vi "Steganography.vi"() -> ()   [LabVIEW 2015]
uses:
  typedefs/_td MainCluster.ctl
  <vilib>/picture/picture.llb/imagedata.ctl
panel:
  in  "_btn Read Text":bool
  out "O_Text":i16[](array[numeric])
  in  "Sigma (decrypt)":i32=2 min=1 max=100
  in  "_btn Stop":bool
  out "Current Operation":string
  out "Current Iteration":i32=10 min=1 max=100
  in  "Repeat N times":i32=1 min=1 max=100
  in  "_btn Process Image":bool
  out "Decrypted Text":string="Some dummy text to build-in."
  in  "Save File Path":path=path "C:/Users/Kosist/Desktop/Megan_processed.bmp"
  in  "Message Energy":dbl=10.0
  in  "Text to Encrypt":string="Lorem ipsum dolor sit amet, consectetur adipiscing elit, sed do eiusmod tempor incididunt ut labore et dolore magna aliqua. Ut enim ad minim veniam, quis nostrud exercitation ullamco laboris nisi ut aliquip ex ea commodo consequat. Duis aute irure dolor in reprehenderit in voluptate velit esse cillum dolore eu fugiat nulla pariatur. Excepteur sint occaecat cupidatat non proident, sunt in culpa qui officia deserunt mollit anim id est laborum."
  in  "Image Path":path=path "C:/Users/Kosist/Desktop/Megan.bmp"
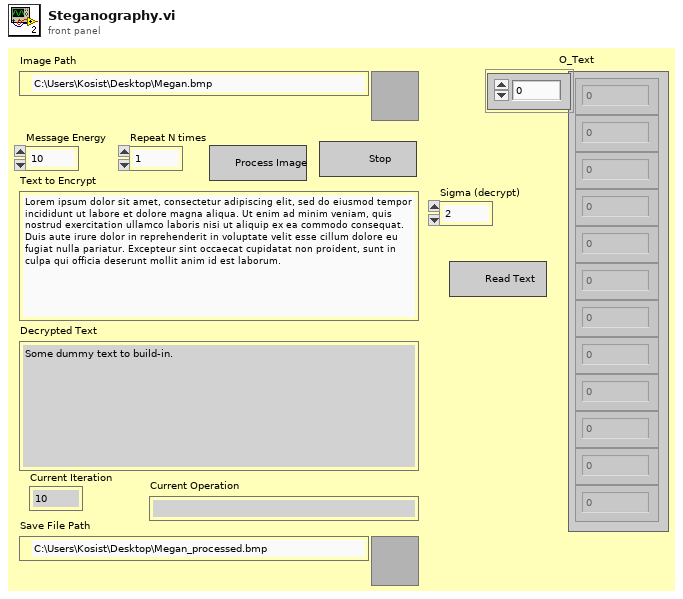
[diagram p1: front panel]
types:
  T1 = enum32{"invalid app kind", "Development System", "Run Time System", "Student Edition", "Embedded LabVIEW", "Evaluation", "Custom"}
  T2 = enum32{"Invalid", "Standard", "Closed", "Hidden", "Minimized", "Maximized"}
  T3 = typedef "_td MainCluster.ctl" = cluster{"SourceImage_FilePath":path, "ProcessedImage_FilePath":path, "Message Energy":dbl, "Text to Encrypt":string, "Decrypted Text":string, "Mixed Pixels Coordinates":i32[][], "Image Data":T4, "Image: Rows":i16, "Image: Columns":i16, "RGB: Red Color":u8[][], "RGB: Green Color":u8[][], "RGB: Blue Color":u8[][], "Required Message Length":i32, "Message Bits Array":u8[], "Mixed RGB Coordinates":i32[], "Repeat N times":i32, "Current Iteration":i32, "Sigma (decrypt)":i32}
  T4 = typedef "imagedata.ctl" = cluster{"image type":i32, "image depth":i32, "image":u8[], "mask":u8[], "colors":u32[], "Rectangle":cluster{"left":i16, "top":i16, "right":i16, "bottom":i16}}
  T5 = cluster{"Core":cluster{"Current VI Reference":refnum<vi>, "Close Panel on Exit?":bool}, "Your Boolean data":bool, "MainCluster":T3}
  T6 = cluster{"Current VI Reference":refnum<vi>, "Close Panel on Exit?":bool}
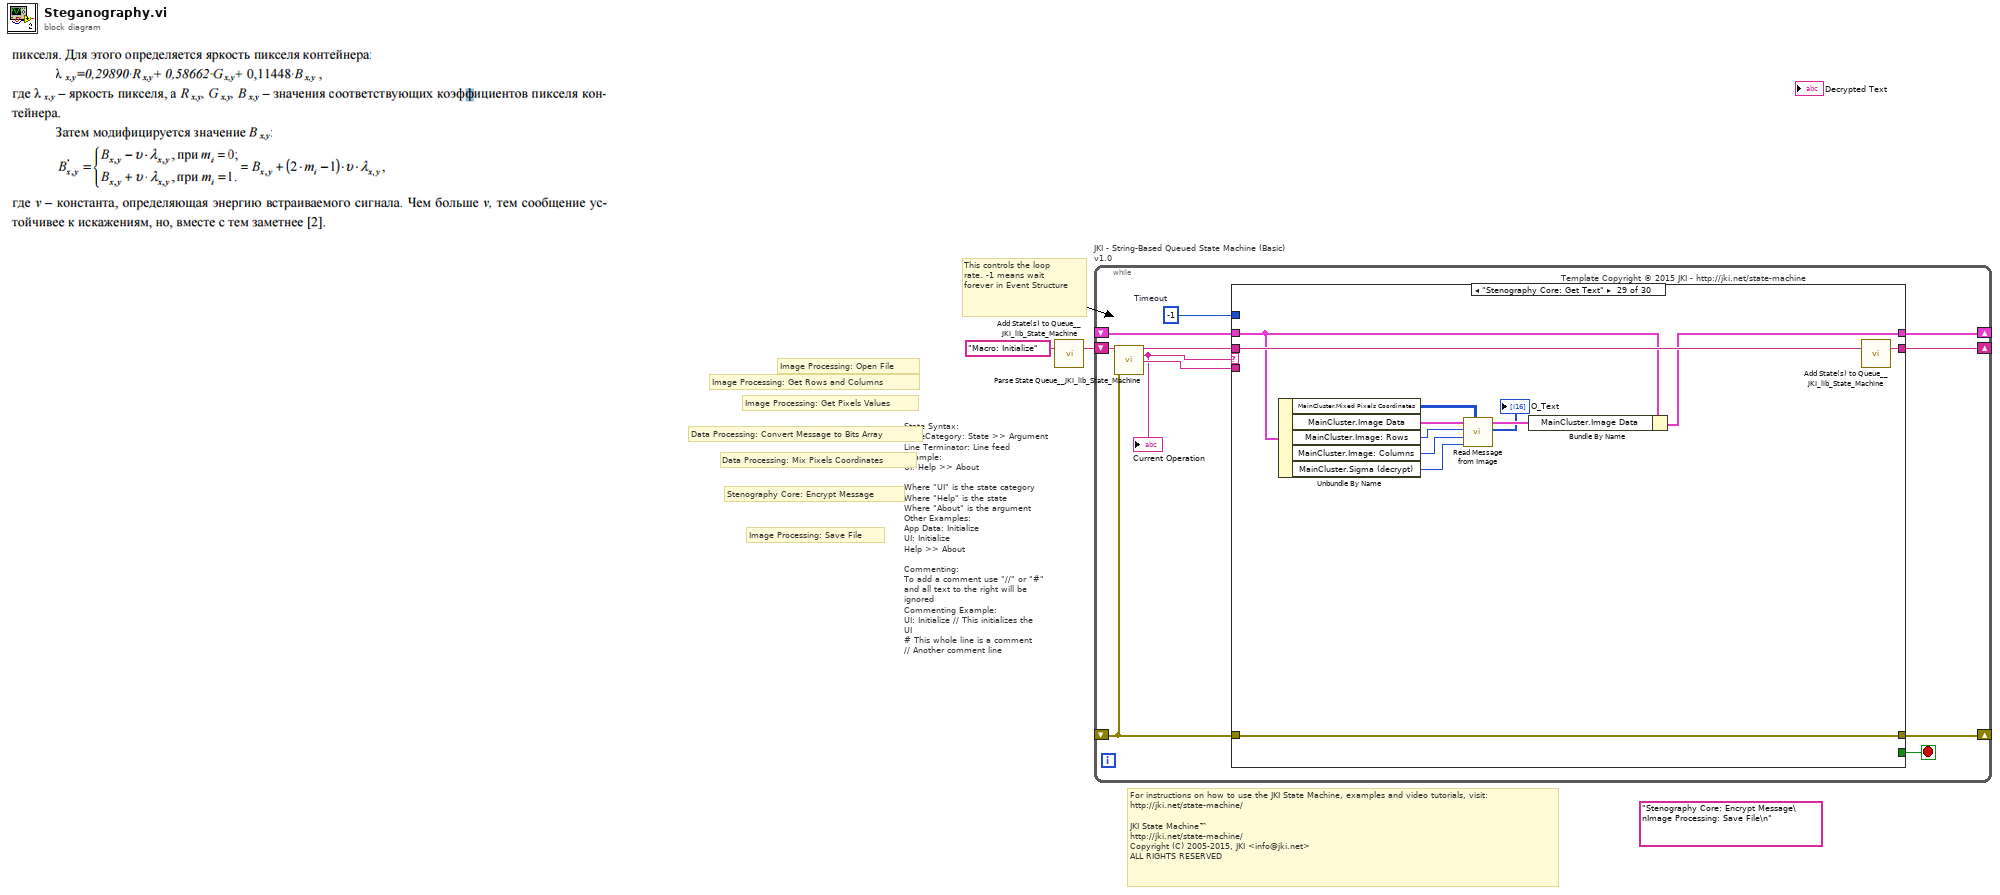
[diagram p0: block diagram]
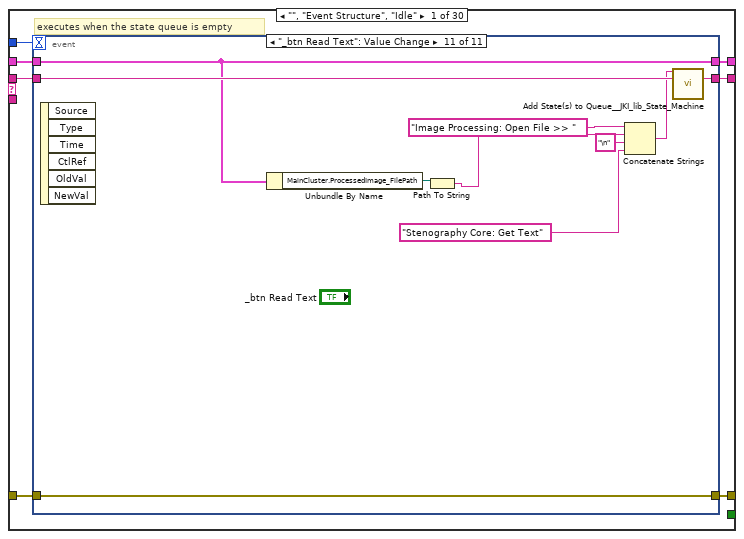
[diagram p2: hidden frame]
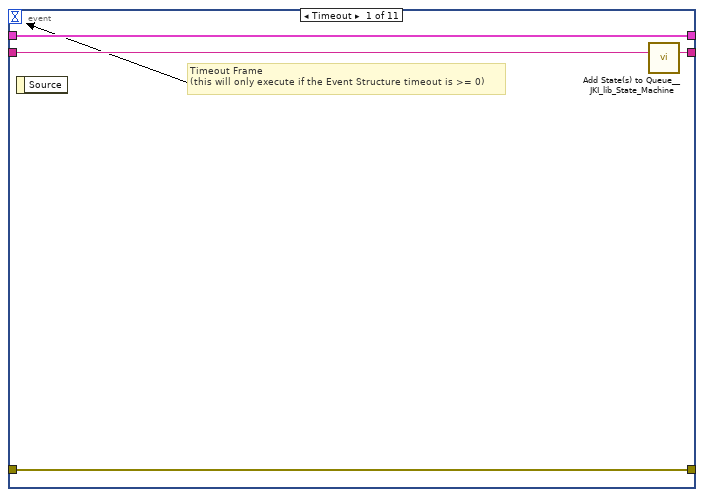
[diagram p3: hidden frame]
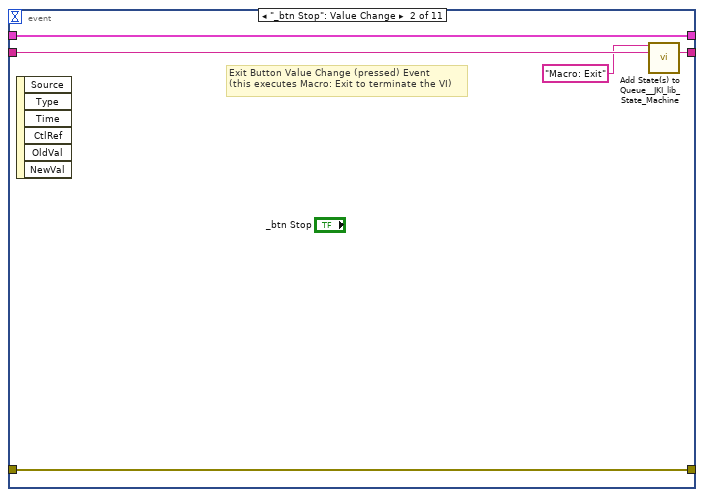
[diagram p4: hidden frame]
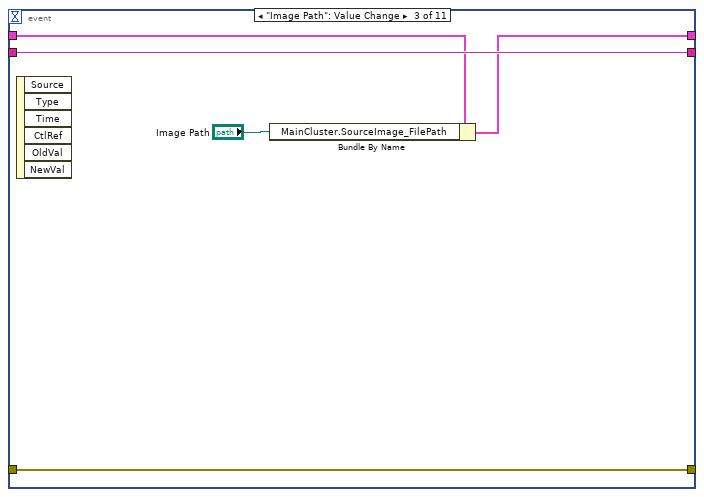
[diagram p5: hidden frame]
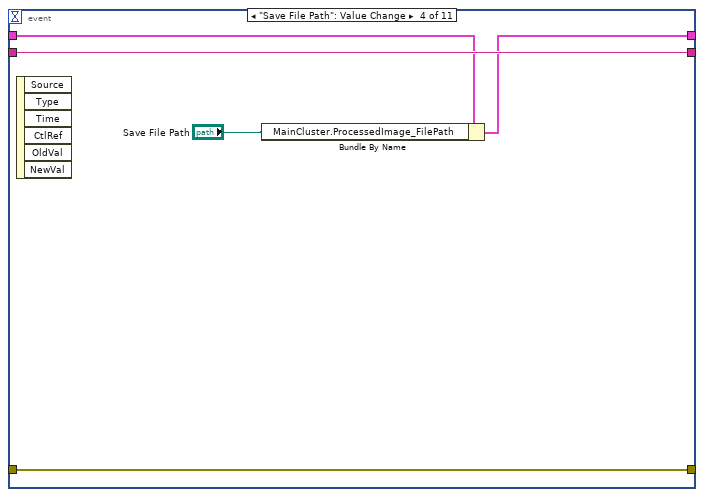
[diagram p6: hidden frame]
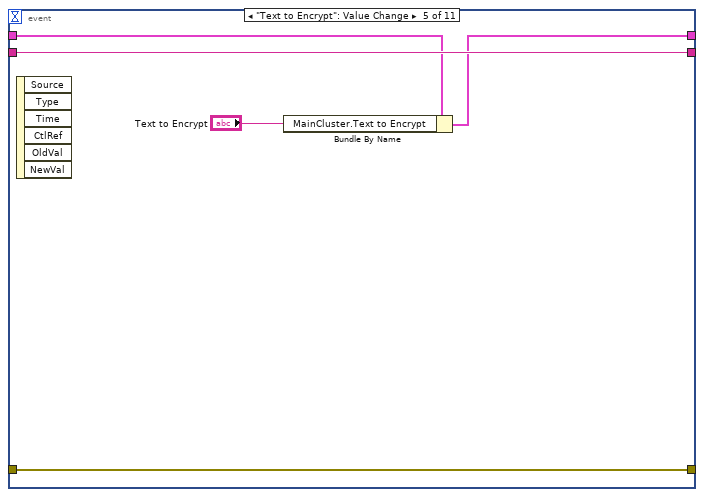
[diagram p7: hidden frame]
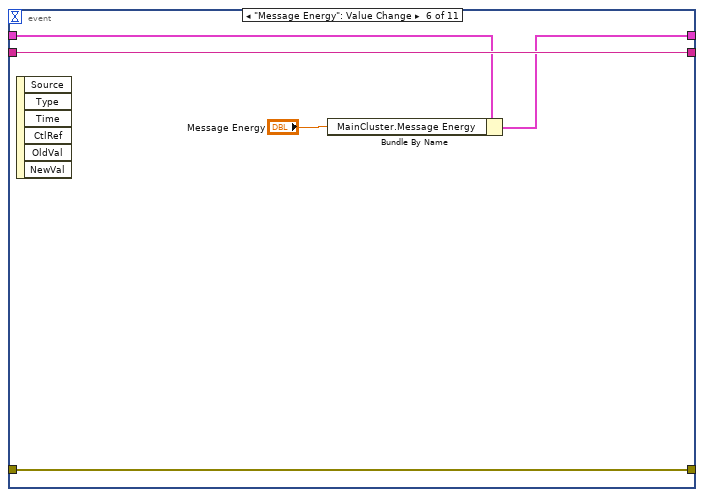
[diagram p8: hidden frame]
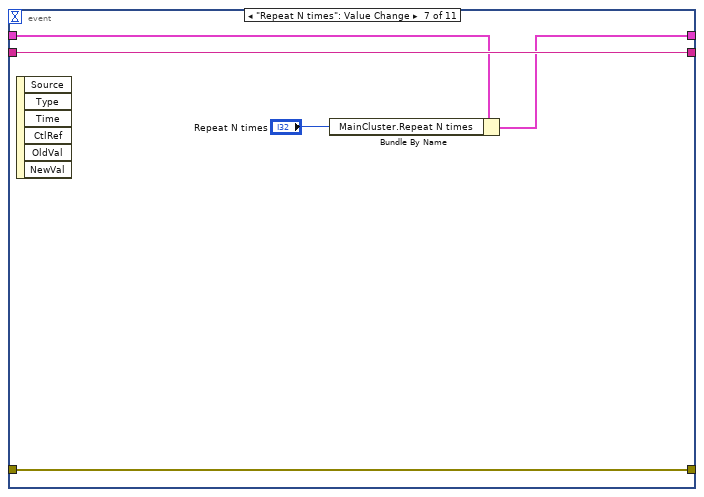
[diagram p9: hidden frame]
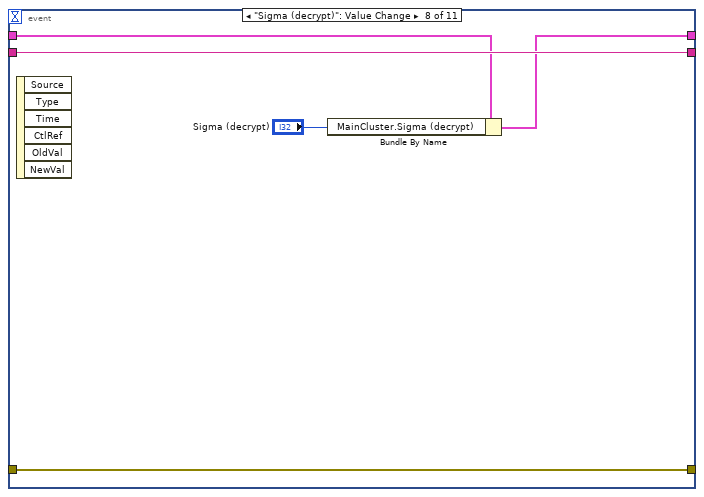
[diagram p10: hidden frame]
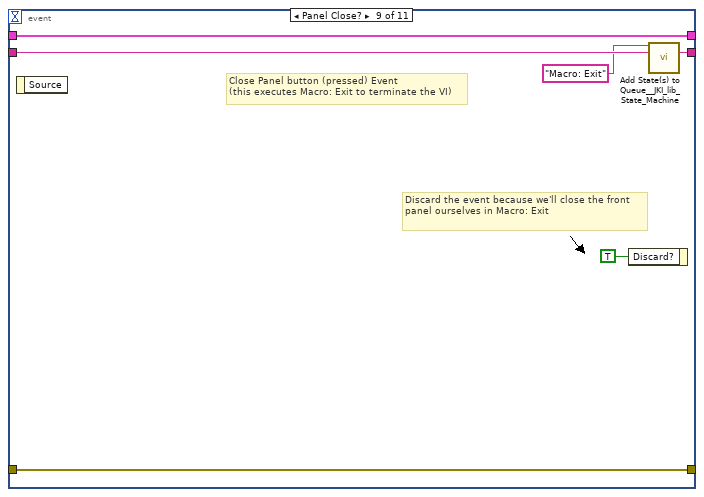
[diagram p11: hidden frame]
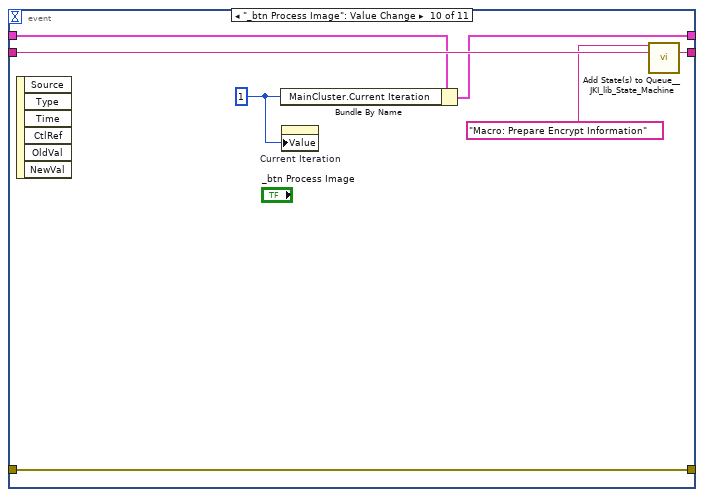
[diagram p12: hidden frame]
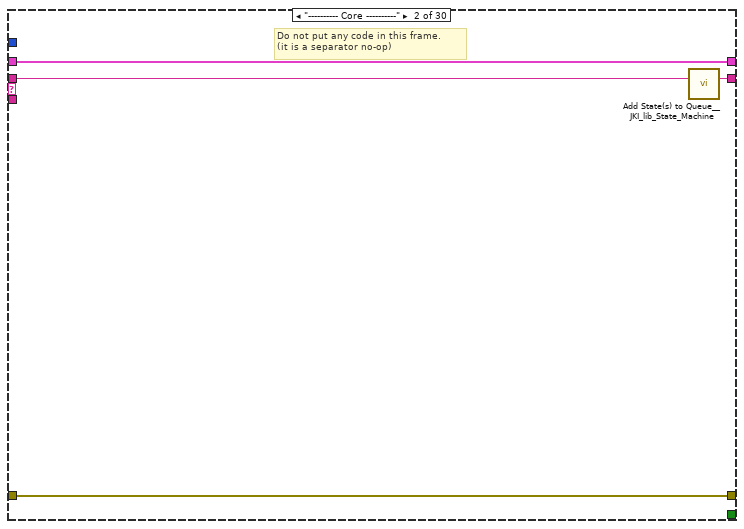
[diagram p13: hidden frame]
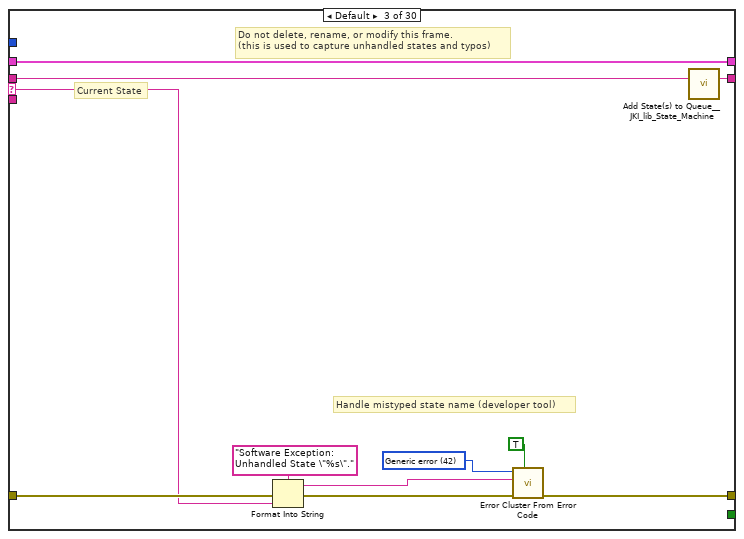
[diagram p14: hidden frame]
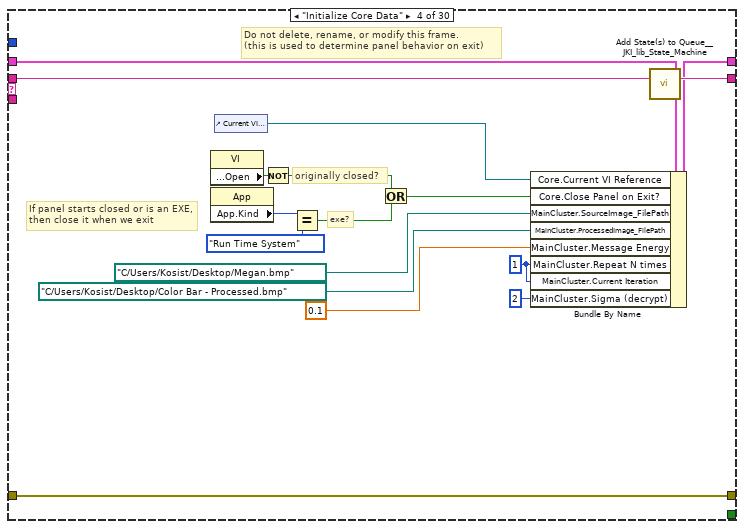
[diagram p15: hidden frame]
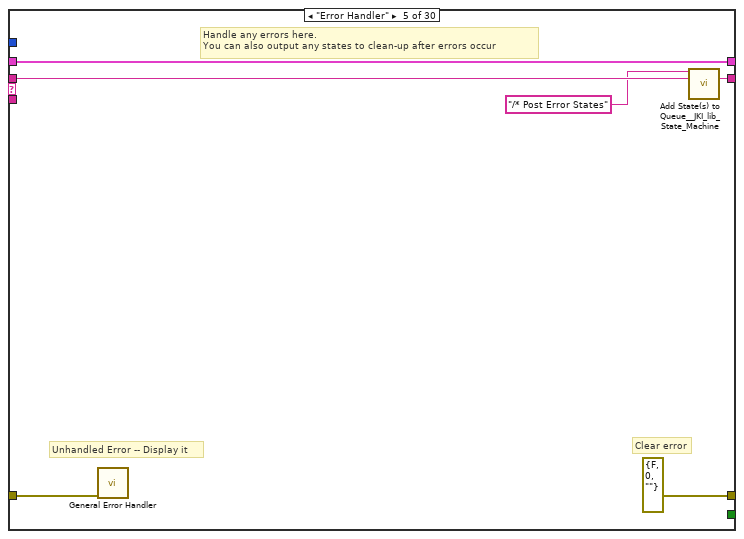
[diagram p16: hidden frame]
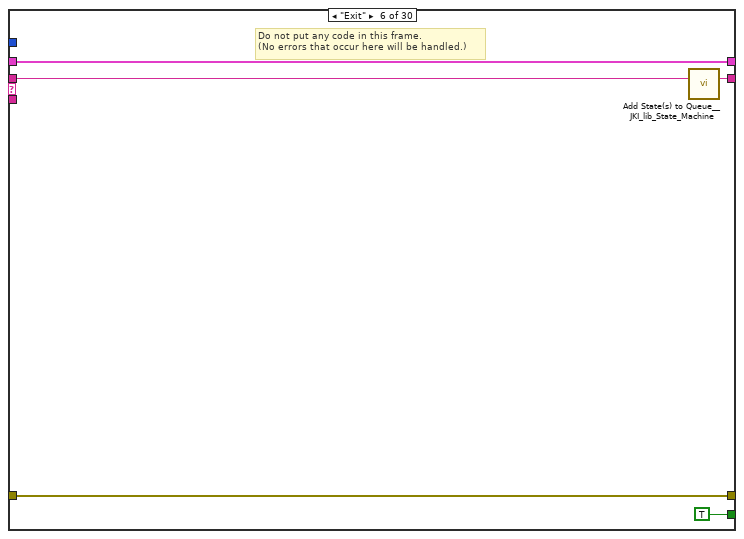
[diagram p17: hidden frame]
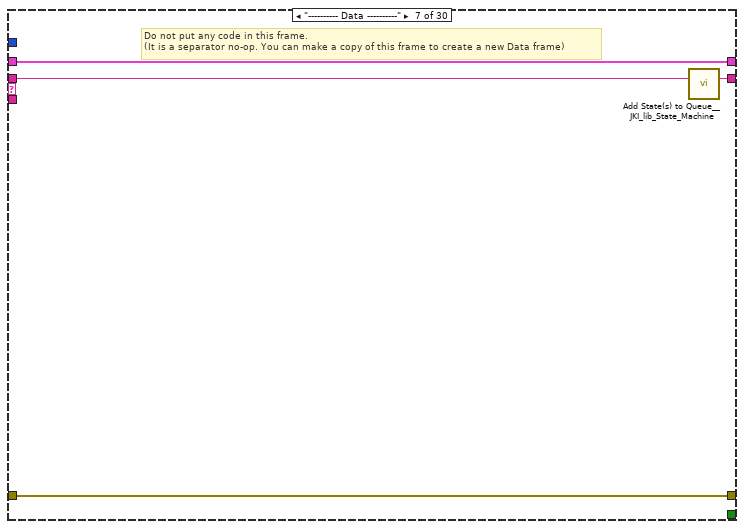
[diagram p18: hidden frame]
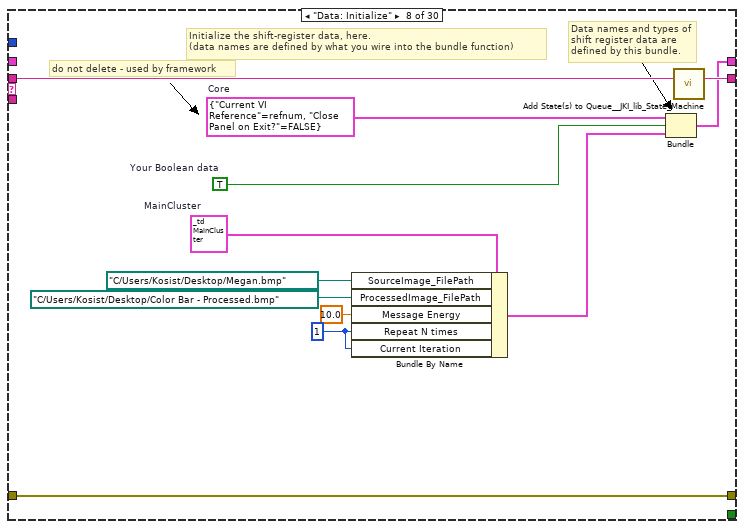
[diagram p19: hidden frame]
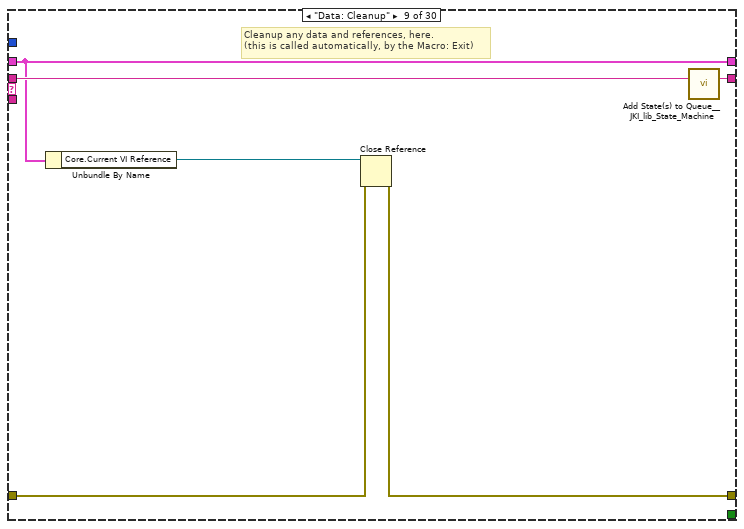
[diagram p20: hidden frame]
diagram:
  (unwired) "Stenography Core: Encrypt Message\nImage Processing: Save File\n"
  # "Image Processing: Save File"
  # "Stenography Core: Encrypt Message"
  # "Data Processing: Mix Pixels Coordinates"
  # "Data Processing: Convert Message to Bits Array"
  # "Image Processing: Get Pixels Values"
  # "Image Processing: Get Rows and Columns"
  # "Image Processing: Open File"
  # "For instructions on how to use the JKI State Machine, examples and video tutorials, visit:\nhttp://jki.net/state-machine/\n\nJKI State Machine™\nhttp://jki.net/state-machine/\nCopyright (C) 2005-2015, JKI <info@jki.net>\nALL RIGHTS RESERVED"
  # "State Syntax:\nStateCategory: State >> Argument\nLine Terminator: Line feed\nExample:\nUI: Help >> About\n\nWhere \"UI\" is the state category\nWhere \"Help\" is the state\nWhere \"About\" is the argument\nOther Examples:\nApp Data: Initialize\nUI: Initialize\nHelp >> About\n\nCommenting:\nTo add a comment use \"//\" or \"#\" and all text to the right will be ignored\nCommenting Example:\nUI: Initialize // This initializes the UI\n# This whole line is a comment\n// Another comment line"
  # "This controls the loop rate. -1 means wait forever in Event Structure"
  n1 = call <vilib>:"Add State(s) to Queue__JKI_lib_State_Machine.vi"("State(s) in (\"\")"="Macro: Initialize") -> ("States Out"=w2:string)  [unwired: 14 in]
  n2 = while "JKI - String-Based Queued State Machine (Basic) v1.0" {
    shift-right: [w7] -> _
    shift-left: _ -> [w6]
    shift-right: [w10] -> _
    shift-left: _ -> [w4]
    shift-right: [w9] -> _
    shift-left: w2 -> [w11]
    stop <- w8 stop-if-true
    w5 = -1  # Timeout
    # "Template Copyright © 2015 JKI - http://jki.net/state-machine"
    n3 = call <vilib>:"Parse State Queue__JKI_lib_State_Machine.vi"("State Queue"=w11, "Error In (no error)"=w4) -> ("Remaining States"=w13:string, "Current State"=w3:string, "Arguments"=w12:string)  [unwired: 11 in]
    "Current Operation" <- w3
    n4 = case shown="\"Stenography Core: Get Text\"" w3 {
      selector: w3 -> [_ _ w87 _ _ _ _ _ _ _ _ _ _ _ _ _ _ _ _ _ _ _ _ _ _ _ _ _ _ _]
      tunnel: w13 -> [w20 w86 w91 w114 w120 w125 w129 w141 w147 w151 w155 w161 w172 w198 w203 w213 w223 w227 w236 w243 w250 w261 w270 w274 w282 w292 w296 w306 w318 w328]
      tunnel: w12 -> [_ _ _ _ _ _ _ _ _ _ _ w156 w166 _ _ _ _ _ w229 _ _ _ _ _ _ _ _ _ _ _]
      tunnel: w6 -> [w18 w83 w89 w105 w117 w123 w126 _ w142 w148 w153 w159 w168 w195 w200 w210 w220 w224 w232 w241 w248 w258 w267 w271 w279 w289 w293 w303 w315 w330]
      tunnel: [w17 w84 w93 w111 errorcluster {"status"=FALSE, "code"=0, "source"=""} ("error out") w122 w127 w138 w143 w149 w152 w157 w169 w196 w201 w211 w221 w225 w233 w237 w247 w259 w268 w272 w280 w290 w294 w304 w316 w319] -> w10
      tunnel: w4 -> [w16 w84 w92 w111 w116 w122 w127 w138 w144 w149 w152 w158 w170 w196 w201 w211 w221 w225 w234 w238 w247 w259 w268 w272 w280 w290 w294 w304 w316 w319]
      tunnel: [w19 w85 w90 w113 w119 w124 w128 w140 w146 w150 w154 w160 w171 w197 w202 w212 w222 w226 w235 w242 w249 w260 w269 w273 w281 w291 w295 w305 w317 w329] -> w9
      tunnel: [_ _ _ _ _ TRUE _ _ _ _ _ _ _ _ _ _ _ _ _ _ _ _ _ _ _ _ _ _ _ _] -> w8
      tunnel: [w15 w83 w89 w112 w117 w123 w126 w139 w142 w148 w153 w159 w168 w195 w200 w210 w220 w224 w231 w241 w246 w257 w266 w271 w278 w285 w293 w298 w314 w326] -> w7
      tunnel: w5 -> [w14 _ _ _ _ _ _ _ _ _ _ _ _ _ _ _ _ _ _ _ _ _ _ _ _ _ _ _ _ _]
      frame "", "Event Structure", "Idle" {
        # "executes when the state queue is empty"
        n5 = event shown="[10] \"_btn Read Text\": Value Change" {
          selector: _ -> [_ _ _ _ _ _ _ _ _ _ _]
          dyn-events: _ -> [_ _ _ _ _ _ _ _ _ _ _]
          timeout: w14 -> [_ _ _ _ _ _ _ _ _ _ _]
          tunnel: w20 -> [w24 w29 w34 w39 w44 w49 w54 w59 w65 w72 w82]
          tunnel: [w23 w28 w34 w39 w44 w49 w54 w59 w64 w71 w81] -> w19
          tunnel: w18 -> [w21 w26 w33 w38 w43 w48 w53 w58 w62 w69 w75]
          tunnel: [w22 w27 w30 w35 w40 w45 w51 w56 w63 w70 w80] -> w17
          tunnel: w16 -> [w22 w27 w30 w35 w40 w45 w51 w56 w63 w70 w80]
          tunnel: [w21 w26 w32 w37 w42 w47 w52 w57 w62 w67 w75] -> w15
          event Timeout {
            # "Timeout Frame\n(this will only execute if the Event Structure timeout is >= 0)"
            n6 = event-data() -> ()  [unwired: 1 in, 1 out]
            n7 = call <vilib>:"Add State(s) to Queue__JKI_lib_State_Machine.vi"("State(s) in (\"\")"=w24) -> ("States Out"=w23:string)  [unwired: 14 in]
          }
          event "_btn Stop": Value Change {
            # "Exit Button Value Change (pressed) Event\n(this executes Macro: Exit to terminate the VI)"
            n8 = event-data() -> ()  [unwired: 1 in, 6 out]
            n9 = call <vilib>:"Add State(s) to Queue__JKI_lib_State_Machine.vi"("State(s) in Front (\"\")"="Macro: Exit", "State(s) in (\"\")"=w29) -> ("States Out"=w28:string)  [unwired: 13 in]
          }
          event "Image Path": Value Change {
            n10 = event-data() -> ()  [unwired: 1 in, 6 out]
            n11 = Bundle By Name(cluster=w33, "MainCluster.SourceImage_FilePath"="Image Path") -> (w32:T5)
          }
          event "Save File Path": Value Change {
            n12 = event-data() -> ()  [unwired: 1 in, 6 out]
            n13 = Bundle By Name(cluster=w38, "MainCluster.ProcessedImage_FilePath"="Save File Path") -> (w37:T5)
          }
          event "Text to Encrypt": Value Change {
            n14 = event-data() -> ()  [unwired: 1 in, 6 out]
            n15 = Bundle By Name(cluster=w43, "MainCluster.Text to Encrypt"="Text to Encrypt") -> (w42:T5)
          }
          event "Message Energy": Value Change {
            n16 = event-data() -> ()  [unwired: 1 in, 6 out]
            n17 = Bundle By Name(cluster=w48, "MainCluster.Message Energy"="Message Energy") -> (w47:T5)
          }
          event "Repeat N times": Value Change {
            n18 = event-data() -> ()  [unwired: 1 in, 6 out]
            n19 = Bundle By Name(cluster=w53, "MainCluster.Repeat N times"="Repeat N times") -> (w52:T5)
          }
          event "Sigma (decrypt)": Value Change {
            n20 = event-data() -> ()  [unwired: 1 in, 6 out]
            n21 = Bundle By Name(cluster=w58, "MainCluster.Sigma (decrypt)"="Sigma (decrypt)") -> (w57:T5)
          }
          event Panel Close? {
            # "Discard the event because we'll close the front panel ourselves in Macro: Exit"
            # "Close Panel button (pressed) Event\n(this executes Macro: Exit to terminate the VI)"
            n22 = event-data() -> ()  [unwired: 1 in, 1 out]
            n23 = event-data("Discard?"=TRUE) -> ()  [unwired: 1 in, 1 out]
            n24 = call <vilib>:"Add State(s) to Queue__JKI_lib_State_Machine.vi"("State(s) in Front (\"\")"="Macro: Exit", "State(s) in (\"\")"=w65) -> ("States Out"=w64:string)  [unwired: 13 in]
          }
          event "_btn Process Image": Value Change {
            w66 = 1 ("MainCluster.Current Iteration")
            n25 = event-data() -> ()  [unwired: 1 in, 6 out]
            n26 = Bundle By Name(cluster=w69, "MainCluster.Current Iteration"=w66) -> (w67:T5)
            n27 = property on="Current Iteration" class="DigNum (strict)"("Value"=w66) -> ()  [unwired: 2 in, 2 out]
            n28 = call <vilib>:"Add State(s) to Queue__JKI_lib_State_Machine.vi"("State(s) in Front (\"\")"="Macro: Prepare Encrypt Information", "State(s) in (\"\")"=w72) -> ("States Out"=w71:string)  [unwired: 13 in]
          }
          event "_btn Read Text": Value Change {
            n29 = event-data() -> ()  [unwired: 1 in, 6 out]
            n30 = Unbundle By Name(w75) -> ("MainCluster.ProcessedImage_FilePath"=w79:path)
            n31 = Path To String(path=w79) -> (string=w77:string)
            n32 = Concatenate Strings("Image Processing: Open File >> ", w77, "\n" ("string"), "Stenography Core: Get Text") -> (w73:string)
            n33 = call <vilib>:"Add State(s) to Queue__JKI_lib_State_Machine.vi"("State(s) in Front (\"\")"=w73, "State(s) in (\"\")"=w82) -> ("States Out"=w81:string)  [unwired: 13 in]
          }
        }
      }
      frame "---------- Core ----------" {
        # "Do not put any code in this frame.\n(it is a separator no-op)"
        n34 = call <vilib>:"Add State(s) to Queue__JKI_lib_State_Machine.vi"("State(s) in (\"\")"=w86) -> ("States Out"=w85:string)  [unwired: 14 in]
      }
      frame Default {
        w96 = 42 items=["No error", "Argument error", "Memory is full", "Out of zone", "End of file", "File already open", "Generic file I/O error", "File not found", "File permission error", "Disk is full", "Duplicate path", "Too many files open", "System feature not enabled", "Resource file not found", "Cannot add resource", "Resource not found", "Image not found", "Image memory error", "Pen does not exist", "Config type invalid", "Config token not found", "Config parse error", "Config memory error", "Bad external code format", "Bad external code offset", "External code not present", "Null window", "Destroy window error", "Null menu", "Print aborted", "Bad print record", "Print driver error", "Windows error during printing", "Memory error during printing", "Print dialog error", "Generic print error", "Invalid device refnum", "Device not found", "Device parameter error", "Device unit error", "Cannot open device", "Device call aborted", "Generic error", "Cancelled by user", "Object ID too low", "Object ID too high", "Object not in heap", "Unknown heap", "Unknown object (invalid DefProc)", "Unknown object (DefProc not in table)", "Message out of range", "Invalid (null) method", "Unknown message", "Manager call not supported", "Bad address", "Network operation in progress", "Network operation timed out", "Connection is busy", "Network attribute not supported", "Network error", "Address in use", "System out of memory", "Connection aborted", "Connection refused", "Not connected", "Already connected", "Connection closed", "Initialization error (interapplication manager)", "Bad occurrence", "Wait on unbound occurrence handler", "Occurrence queue overflow", "Datalog type conflict", "Unused", "Unrecognized type (interapplication manager)", "Memory corrupt", "Failed to make temporary DLL", "Old CIN version", "Drag socket not found", "Failed to load drop-object", "Failed to register OLE object", "Failed to release OLE object", "Format specifier type mismatch", "Unknown format specifier", "Too few format specifiers", "Too many format specifiers", "Scan failed", "Newer CIN version", "Error converting to variant", "Runtime menu error", "Password tampered", "Variant attribute not found", "Incompatible variant data type", "Event data is not available", "Event Store is not present", "Occurrence is not found", "Event Queue is not created", "Event info is not available", "Refnum passed is NULL", "Error retrieving Class GUID", "Error retrieving CoClass GUID", "Error retrieving TypeLib GUID.", "Bad built application magic bytes.", "Specific driver is different from the specific driver associated with the Logical Name.", "There is no session opened to the class driver.", "Max Error", "MAX - Error with config objects", "MAX - Error loading configuration", "MAX - Group not supported"]
        # "Current State"
        # "Do not delete, rename, or modify this frame.\n(this is used to capture unhandled states and typos)"
        # "Handle mistyped state name (developer tool)"
        n35 = Format Into String(format string="Software Exception: Unhandled State \"%s\"." ("message"), error in=w92, w87) -> (resulting string=w95:string, error out=w94:errorcluster)  [unwired: 1 in]
        n36 = call <vilib>:"Error Cluster From Error Code.vi"("show call chain? (False)"=TRUE, "error in (no error)"=w94, "error message (\"\")"=w95, "error code (0)"=w96) -> ("error out"=w93:errorcluster)  [unwired: 5 in]
        n37 = call <vilib>:"Add State(s) to Queue__JKI_lib_State_Machine.vi"("State(s) in (\"\")"=w91) -> ("States Out"=w90:string)  [unwired: 14 in]
      }
      frame "Initialize Core Data" {
        w99 = 1 ("MainCluster.Repeat N times")
        # "Do not delete, rename, or modify this frame.\n(this is used to determine panel behavior on exit)"
        # "originally closed?"
        # "exe?"
        # "If panel starts closed or is an EXE, then close it when we exit"
        n38 = property class="VI"() -> ("Front Panel.Open"=w110:bool)  [unwired: 2 in, 2 out]
        n39 = property class="App"() -> ("App.Kind"=w109:T1)  [unwired: 2 in, 2 out]
        n40 = control-ref of="Current VI Reference"() -> (w103:refnum<vi>)
        n41 = Not(x=w110) -> (.not. x?=w107:bool)
        n42 = Equal?(x=w109, y=T1."Run Time System" ("Application:Kind")) -> (x = y?=w106:bool)
        n43 = Or(x=w107, y=w106) -> (x .or. y?=w104:bool)
        n44 = Bundle By Name(cluster=w105, "Core.Current VI Reference"=w103, "Core.Close Panel on Exit?"=w104, "MainCluster.SourceImage_FilePath"=path "C:/Users/Kosist/Desktop/Megan.bmp" ("_td MainCluster.SourceImage_FilePath"), "MainCluster.ProcessedImage_FilePath"=path "C:/Users/Kosist/Desktop/Color Bar - Processed.bmp" ("_td MainCluster.SourceImage_FilePath"), "MainCluster.Message Energy"=0.1 ("_td MainCluster.Message Energy"), "MainCluster.Repeat N times"=w99, "MainCluster.Current Iteration"=w99, "MainCluster.Sigma (decrypt)"=2) -> (w112:T5)
        n45 = call <vilib>:"Add State(s) to Queue__JKI_lib_State_Machine.vi"("State(s) in (\"\")"=w114) -> ("States Out"=w113:string)  [unwired: 14 in]
      }
      frame "Error Handler" {
        # "Unhandled Error -- Display it"
        # "Handle any errors here.\nYou can also output any states to clean-up after errors occur"
        # "Clear error"
        n46 = call <vilib>:"General Error Handler.vi"("error in (no error)"=w116) -> ()  [unwired: 10 in, 5 out]
        n47 = call <vilib>:"Add State(s) to Queue__JKI_lib_State_Machine.vi"("State(s) in Front (\"\")"="/* Post Error States", "State(s) in (\"\")"=w120) -> ("States Out"=w119:string)  [unwired: 13 in]
      }
      frame "Exit" {
        # "Do not put any code in this frame.\n(No errors that occur here will be handled.)"
        n48 = call <vilib>:"Add State(s) to Queue__JKI_lib_State_Machine.vi"("State(s) in (\"\")"=w125) -> ("States Out"=w124:string)  [unwired: 14 in]
      }
      frame "---------- Data ----------" {
        # "Do not put any code in this frame.\n(It is a separator no-op. You can make a copy of this frame to create a new Data frame)"
        n49 = call <vilib>:"Add State(s) to Queue__JKI_lib_State_Machine.vi"("State(s) in (\"\")"=w129) -> ("States Out"=w128:string)  [unwired: 14 in]
      }
      frame "Data: Initialize" {
        w130 = 1 ("Repeat N times")
        w135 = T3 {"SourceImage_FilePath"=path "", "ProcessedImage_FilePath"=path "", "Message Energy"=0.0, "Text to Encrypt"="", "Decrypted Text"="", "Mixed Pixels Coordinates"=[], "Image Data"={"image type"=0, "image depth"=0, "image"=[], "mask"=[], "colors"=[], "Rectangle"={"left"=0, "top"=0, "right"=0, "bottom"=0}}, "Image: Rows"=0, "Image: Columns"=0, "RGB: Red Color"=[], "RGB: Green Color"=[], "RGB: Blue Color"=[], "Required Message Length"=0, "Message Bits Array"=[], "Mixed RGB Coordinates"=[], "Repeat N times"=0, "Current Iteration"=0, "Sigma (decrypt)"=2}  # MainCluster
        w136 = T6 {"Current VI Reference"=refnum, "Close Panel on Exit?"=FALSE}  # Core
        w137 = TRUE  # Your Boolean data
        # "do not delete - used by framework"
        # "Data names and types of shift register data are defined by this bundle."
        # "Initialize the shift-register data, here.\n(data names are defined by what you wire into the bundle function)"
        n50 = Bundle By Name(cluster=w135, "SourceImage_FilePath"=path "C:/Users/Kosist/Desktop/Megan.bmp" ("Image Path"), "ProcessedImage_FilePath"=path "C:/Users/Kosist/Desktop/Color Bar - Processed.bmp" ("Save File Path"), "Message Energy"=10.0, "Repeat N times"=w130, "Current Iteration"=w130) -> (w134:T3)
        n51 = Bundle("Core"=w136, "Your Boolean data"=w137, "MainCluster"=w134) -> (w139:T5)  [unwired: 1 in]
        n52 = call <vilib>:"Add State(s) to Queue__JKI_lib_State_Machine.vi"("State(s) in (\"\")"=w141) -> ("States Out"=w140:string)  [unwired: 14 in]
      }
      frame "Data: Cleanup" {
        # "Cleanup any data and references, here.\n(this is called automatically, by the Macro: Exit)"
        n53 = Unbundle By Name(w142) -> ("Core.Current VI Reference"=w145:refnum<vi>)
        n54 = Close Reference(reference=w145, error in (no error)=w144) -> (error out=w143:errorcluster)
        n55 = call <vilib>:"Add State(s) to Queue__JKI_lib_State_Machine.vi"("State(s) in (\"\")"=w147) -> ("States Out"=w146:string)  [unwired: 14 in]
      }
      frame "---------- UI ----------" {
        # "Do not put any code in this frame.\n(It is a separator no-op. You can make a copy of this frame to create a new UI frame)"
        n56 = call <vilib>:"Add State(s) to Queue__JKI_lib_State_Machine.vi"("State(s) in (\"\")"=w151) -> ("States Out"=w150:string)  [unwired: 14 in]
      }
      frame "UI: Initialize" {
        # "Initialize the User Interface, here.\n(this is called automatically, by the Macro: Init)"
        n57 = call <vilib>:"Add State(s) to Queue__JKI_lib_State_Machine.vi"("State(s) in (\"\")"=w155) -> ("States Out"=w154:string)  [unwired: 14 in]
      }
      frame "UI: Cursor Set" {
        # "Argument"
        # "Set and Unset Cursor Busy.\n(Usage: \"UI: Cursor Set >> Busy|Idle\")"
        n58 = case shown="\"Idle\", Default" w156 {
          tunnel: w158 -> [w163 w165]
          tunnel: [w162 w164] -> w157
          frame "Idle", Default {
            n59 = call <vilib>:"Unset Busy.vi"("error in (no error)"=w163) -> ("error out"=w162:errorcluster)  [unwired: 10 in]
          }
          frame "Busy" {
            n60 = call <vilib>:"Set Busy.vi"("error in (no error)"=w165) -> ("error out"=w164:errorcluster)  [unwired: 9 in, 1 out]
          }
        }
        n61 = call <vilib>:"Add State(s) to Queue__JKI_lib_State_Machine.vi"("State(s) in (\"\")"=w161) -> ("States Out"=w160:string)  [unwired: 14 in]
      }
      frame "UI: Front Panel State" {
        # "Argument"
        # "Set Front Panel Open or Closed\n(Usage: \"UI: Front Panel State >> Open|Close\")"
        n62 = Unbundle By Name(w168) -> ("Core.Current VI Reference"=w167:refnum<vi>)
        n63 = case shown="\"Open\", Default" w166 {
          tunnel: w170 -> [w176 w189]
          tunnel: [w178 w190] -> w169
          tunnel: w167 -> [w177 w187]
          frame "Open", Default {
            n64 = property class="VI"(reference=w177, error in=w176) -> (reference out=w174:refnum<vi>, error out=w175:errorcluster, "Front Panel.Open"=w173:bool)
            n65 = case shown="False" w173 {
              tunnel: [w181 w184] -> w178
              tunnel: w175 -> [w180 w184]
              tunnel: w174 -> [w179 _]
              frame False {
                n66 = invoke class="VI" method="FP.Open"(reference=w179, error in=w180, "Activate"=TRUE, "State"=T2."Standard") -> (error out=w181:errorcluster)  [unwired: 1 in, 4 out]
              }
              frame True {
              }
            }
          }
          frame "Close" {
            n67 = property class="VI"(reference=w187, error in=w189) -> (reference out=w186:refnum<vi>, error out=w188:errorcluster, "Front Panel.Open"=w185:bool)
            n68 = case shown="True" w185 {
              tunnel: [w191 w194] -> w190
              tunnel: w188 -> [w191 w193]
              tunnel: w186 -> [_ w192]
              frame False {
              }
              frame True {
                n69 = invoke class="VI" method="FP.Close"(reference=w192, error in=w193) -> (error out=w194:errorcluster)  [unwired: 1 in, 2 out]
              }
            }
          }
        }
        n70 = call <vilib>:"Add State(s) to Queue__JKI_lib_State_Machine.vi"("State(s) in (\"\")"=w172) -> ("States Out"=w171:string)  [unwired: 14 in]
      }
      frame "---------- Macro ----------" {
        # "Do not put any code in this frame.\n(It is a separator no-op. You can make a copy of this frame to create a new Macro frame)"
        n71 = call <vilib>:"Add State(s) to Queue__JKI_lib_State_Machine.vi"("State(s) in (\"\")"=w198) -> ("States Out"=w197:string)  [unwired: 14 in]
      }
      frame "Macro: Initialize" {
        w199 = "Data: Initialize\nInitialize Core Data\nUI: Initialize\nUI: Front Panel State >> Open"  # Data: Initialize Initialize Core Data UI: Initialize UI: Front Panel State >> Open
        # "Initialization Macro\n(This is called once, when the VI starts)"
        n72 = call <vilib>:"Add State(s) to Queue__JKI_lib_State_Machine.vi"("State(s) in Front (\"\")"=w199, "State(s) in (\"\")"=w203) -> ("States Out"=w202:string)  [unwired: 13 in]
      }
      frame "Macro: Prepare Encrypt Information" {
        n73 = Unbundle By Name(w210) -> ("MainCluster.SourceImage_FilePath"=w209:path)
        n74 = Path To String(path=w209) -> (string=w207:string)
        n75 = Concatenate Strings("Image Processing: Open File >> ", w207, "\n" ("string"), "Image Processing: Get Rows and Columns\nImage Processing: Get Pixels Values\nData Processing: Convert Message to Bits Array\nData Processing: Mix Pixels Coordinates\nStenography Core: Encrypt Message\nStenography Core: Iteration Control") -> (w204:string)
        n76 = call <vilib>:"Add State(s) to Queue__JKI_lib_State_Machine.vi"("State(s) in Front (\"\")"=w204, "State(s) in (\"\")"=w213) -> ("States Out"=w212:string)  [unwired: 13 in]
      }
      frame "Macro: Exit" {
        # "Exit Macro\n(This is called once, when the VI exits)"
        n77 = Unbundle By Name(w220) -> ("Core.Close Panel on Exit?"=w219:bool)
        n78 = Select(t="UI: Front Panel State >> Close", s=w219, f="") -> (s? t:f=w216:string)
        n79 = call <vilib>:"Add State(s) to Queue__JKI_lib_State_Machine.vi"("State(s) in (\"\")"=w216, "State(s) at Back (\"\")"="Data: Cleanup\nExit") -> ("States Out"=w214:string)  [unwired: 13 in]
        n80 = call <vilib>:"Add State(s) to Queue__JKI_lib_State_Machine.vi"("State(s) in Front (\"\")"=w214, "State(s) in (\"\")"=w223) -> ("States Out"=w222:string)  [unwired: 13 in]
      }
      frame "---------- Image Processing ----------" {
        # "Template Separator\n(You can make a copy of, or modify, this frame)"
        n81 = call <vilib>:"Add State(s) to Queue__JKI_lib_State_Machine.vi"("State(s) in (\"\")"=w227) -> ("States Out"=w226:string)  [unwired: 14 in]
      }
      frame "Image Processing: Open File" {
        n82 = String To Path(string=w229) -> (path=w228:path)
        n83 = call <vilib>:"Read BMP File.vi"("error in (no error)"=w234, "path to BMP file"=w228) -> ("error out"=w233:errorcluster, "image data"=w230:T4)  [unwired: 7 in, 1 out]
        n84 = Bundle By Name(cluster=w232, "MainCluster.Image Data"=w230) -> (w231:T5)
        n85 = call <vilib>:"Add State(s) to Queue__JKI_lib_State_Machine.vi"("State(s) in (\"\")"=w236) -> ("States Out"=w235:string)  [unwired: 14 in]
      }
      frame "Image Processing: Save File" {
        n86 = Unbundle By Name(w241) -> ("MainCluster.ProcessedImage_FilePath"=w240:path, "MainCluster.Image Data"=w239:T4)
        n87 = call <vilib>:"Write BMP File.vi"("error in (no error)"=w238, "image data"=w239, "path to BMP file"=w240) -> ("error out"=w237:errorcluster)  [unwired: 7 in, 1 out]
        n88 = call <vilib>:"Add State(s) to Queue__JKI_lib_State_Machine.vi"("State(s) in (\"\")"=w243) -> ("States Out"=w242:string)  [unwired: 14 in]
      }
      frame "Image Processing: Get Rows and Columns" {
        n89 = Unbundle By Name(w248) -> ("MainCluster.Image Data.Rectangle.bottom"=w245:i16, "MainCluster.Image Data.Rectangle.right"=w244:i16)
        n90 = Bundle By Name(cluster=w248, "MainCluster.Image: Rows"=w245, "MainCluster.Image: Columns"=w244) -> (w246:T5)
        n91 = call <vilib>:"Add State(s) to Queue__JKI_lib_State_Machine.vi"("State(s) in (\"\")"=w250) -> ("States Out"=w249:string)  [unwired: 14 in]
      }
      frame "Image Processing: Get Pixels Values" {
        n92 = Unbundle By Name(w258) -> ("MainCluster.Image Data.image"=w256:u8[], "MainCluster.Image Data.Rectangle.bottom"=w255:i16, "MainCluster.Image Data.Rectangle.right"=w254:i16)
        n93 = call "Get RGB Pixels Values.vi"("I_Number of columns"=w254, "I_Number of rows"=w255, "I_Image Data"=w256) -> ("O_RGB: Blue Color"=w251:u8[][], "O_RGB: Green Color"=w252:u8[][], "O_RGB: Red Color"=w253:u8[][])  [unwired: 6 in]
        n94 = Bundle By Name(cluster=w258, "MainCluster.RGB: Red Color"=w253, "MainCluster.RGB: Green Color"=w252, "MainCluster.RGB: Blue Color"=w251) -> (w257:T5)
        n95 = call <vilib>:"Add State(s) to Queue__JKI_lib_State_Machine.vi"("State(s) in (\"\")"=w261) -> ("States Out"=w260:string)  [unwired: 14 in]
      }
      frame "Image Processing: Pixels Values to Image" {
        n96 = Unbundle By Name(w267) -> ("MainCluster.RGB: Red Color"=w265:u8[][], "MainCluster.RGB: Green Color"=w264:u8[][], "MainCluster.RGB: Blue Color"=w263:u8[][])
        n97 = call "RGB Pixels Values to Image.vi"("I_RGB: Blue Color"=w263, "I_RGB: Green Color"=w264, "I_RGB: Red Color"=w265) -> ("O_Image Data"=w262:u8[])  [unwired: 8 in]
        n98 = Bundle By Name(cluster=w267, "MainCluster.Image Data.image"=w262) -> (w266:T5)
        n99 = call <vilib>:"Add State(s) to Queue__JKI_lib_State_Machine.vi"("State(s) in (\"\")"=w270) -> ("States Out"=w269:string)  [unwired: 14 in]
      }
      frame "---------- Data Processing ----------" {
        # "Template Separator\n(You can make a copy of, or modify, this frame)"
        n100 = call <vilib>:"Add State(s) to Queue__JKI_lib_State_Machine.vi"("State(s) in (\"\")"=w274) -> ("States Out"=w273:string)  [unwired: 14 in]
      }
      frame "Data Processing: Convert Message to Bits Array" {
        n101 = Unbundle By Name(w279) -> ("MainCluster.Text to Encrypt"=w277:string)
        n102 = call "Convert String to Bits Array.vi"("I_String"=w277) -> ("O_Bits Array"=w275:i16[])  [unwired: 10 in]
        n103 = Array Size(array=w275) -> (size(s)=w276:i32)
        n104 = Bundle By Name(cluster=w279, "MainCluster.Message Bits Array"=w275, "MainCluster.Required Message Length"=w276) -> (w278:T5)
        n105 = call <vilib>:"Add State(s) to Queue__JKI_lib_State_Machine.vi"("State(s) in (\"\")"=w282) -> ("States Out"=w281:string)  [unwired: 14 in]
      }
      frame "Data Processing: Mix Pixels Coordinates" {
        n106 = Unbundle By Name(w289) -> ("MainCluster.Image: Rows"=w288:i16, "MainCluster.Image: Columns"=w287:i16, "MainCluster.Required Message Length"=w286:i32)
        n107 = call "Mix Coordinates Array.vi"("I_Required Length"=w286, "I_Number of columns"=w287, "I_Number of rows"=w288) -> ("O_Mixed RGB Coordinates"=w283:i32[], "O_Mixed Coordinates"=w284:i32[][])  [unwired: 7 in]
        n108 = Bundle By Name(cluster=w289, "MainCluster.Mixed Pixels Coordinates"=w284, "MainCluster.Mixed RGB Coordinates"=w283) -> (w285:T5)
        n109 = call <vilib>:"Add State(s) to Queue__JKI_lib_State_Machine.vi"("State(s) in (\"\")"=w292) -> ("States Out"=w291:string)  [unwired: 14 in]
      }
      frame "---------- Stenography Core ----------" {
        # "Template Separator\n(You can make a copy of, or modify, this frame)"
        n110 = call <vilib>:"Add State(s) to Queue__JKI_lib_State_Machine.vi"("State(s) in (\"\")"=w296) -> ("States Out"=w295:string)  [unwired: 14 in]
      }
      frame "Stenography Core: Encrypt Message" {
        n111 = Unbundle By Name(w303) -> ("MainCluster.Image Data"=w302:T4, "MainCluster.Message Energy"=w301:dbl, "MainCluster.Message Bits Array"=w300:u8[], "MainCluster.Mixed RGB Coordinates"=w299:i32[])
        n112 = call "Write Message to Image.vi"("I_Mixed RGB Coordinates"=w299, "I_Message Bits to Code"=w300, "I_Message Energy"=w301, "I_Image Data"=w302) -> ("O_Image Data"=w297:T4)  [unwired: 7 in]
        n113 = Bundle By Name(cluster=w303, "MainCluster.Image Data"=w297) -> (w298:T5)
        n114 = call <vilib>:"Add State(s) to Queue__JKI_lib_State_Machine.vi"("State(s) in (\"\")"=w306) -> ("States Out"=w305:string)  [unwired: 14 in]
      }
      frame "Stenography Core: Get Text" {
        n115 = Unbundle By Name(w315) -> ("MainCluster.Mixed Pixels Coordinates"=w311:i32[][], "MainCluster.Image Data"=w313:T4, "MainCluster.Image: Rows"=w310:i16, "MainCluster.Image: Columns"=w309:i16, "MainCluster.Sigma (decrypt)"=w308:i32)
        n116 = call "Read Message from Image.vi"("I_Mixed Coordinates"=w311, "I_Sigma"=w308, "I_Number of columns"=w309, "I_Number of rows"=w310, "I_Image Data"=w313) -> ("O_Text"=→"O_Text":i16[], "O_Image Data"=w312:T4)  [unwired: 5 in]
        n117 = Bundle By Name(cluster=w315, "MainCluster.Image Data"=w312) -> (w314:T5)
        n118 = call <vilib>:"Add State(s) to Queue__JKI_lib_State_Machine.vi"("State(s) in (\"\")"=w318) -> ("States Out"=w317:string)  [unwired: 14 in]
      }
      frame "Stenography Core: Iteration Control" {
        n119 = Unbundle By Name(w330) -> ("MainCluster.Repeat N times"=w327:i32, "MainCluster.Current Iteration"=w321:i32)
        n120 = Greater?(x=w327, y=w321) -> (0:w325:bool)
        n121 = Select(t="Stenography Core: Encrypt Message\nStenography Core: Iteration Control", s=w325, f="Image Processing: Save File") -> (s? t:f=w322:string)
        n122 = Increment(x=w321) -> (x+1=w320:i32)
        "Current Iteration" <- w320
        n123 = Bundle By Name(cluster=w330, "MainCluster.Current Iteration"=w320) -> (w326:T5)
        n124 = call <vilib>:"Add State(s) to Queue__JKI_lib_State_Machine.vi"("State(s) in (\"\")"=w328, "State(s) at Back (\"\")"=w322) -> ("States Out"=w329:string)  [unwired: 13 in]
      }
    }
  }
